vi "Test Pickup Tool Load.vi"() -> ()   [LabVIEW 2011]
uses:
  PickupTool Class.lvclass
  Gantry Class/Gantry Class.lvclass
panel:
  out "error out":errorcluster
  in  "Config Folder":path=path "C:/Users/Husker/Desktop/gantry/Config"
  in  "HOME?":bool
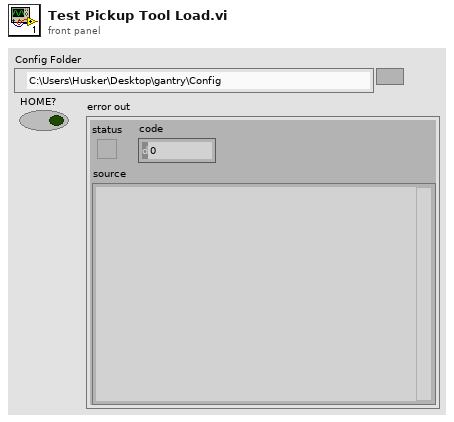
[diagram p1: front panel]
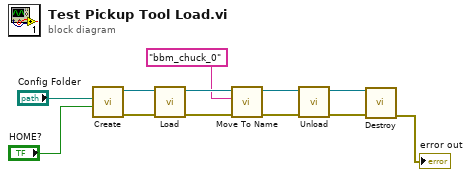
[diagram p0: block diagram]
diagram:
  n1 = call "Create.vi"("HOME?"="HOME?", "Config Folder"="Config Folder") -> ("error out"=w9:errorcluster, "Gantry out"=w10:refnum<class "Gantry Class.lvclass">)  [unwired: 8 in]
  n2 = call "Load.vi"("error in"=w9, "Gantry in"=w10) -> ("error out"=w7:errorcluster, "PickupTool out"=w8:refnum<class "PickupTool Class.lvclass">)  [unwired: 8 in]
  n3 = call-dynamic "Move To Name.vi"("error in"=w7, "Destination Name"="bbm_chuck_0", "Gantry in"=w8) -> ("error out"=w4:errorcluster, "Gantry out"=w5:refnum<class "PickupTool Class.lvclass">)  [unwired: 7 in]
  n4 = call "Unload.vi"("error in"=w4, "PickupTool in"=w5) -> ("error out"=w2:errorcluster, "Gantry out"=w3:refnum<class "Gantry Class.lvclass">)  [unwired: 8 in]
  n5 = call "Destroy.vi"("error in"=w2, "Gantry Class in"=w3) -> ("error out"=→"error out":errorcluster)  [unwired: 9 in]
